vi "Instrument Manager_CleanUp.vi"(8 "Error In":errorcluster) -> (0 "Error Out":errorcluster)   [LabVIEW 2024, in "Instrument Manager.lvclass"]
uses:
  Instrument Manager.lvclass
  Interfaces/IUnmanaged/IUnmanaged.lvclass
  Interfaces/IInstrument/IInstrument.lvclass
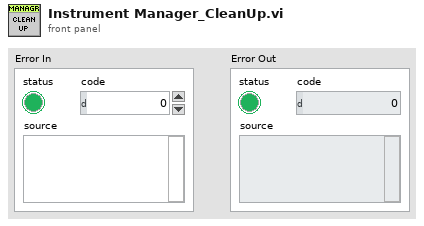
[diagram p1: front panel]
types:
  T1 = typedef "Instrument Manager.lvclass/ObjectAttributes.ctl" = cluster{"IInstruments":map{string, refnum<class "IInstrument.lvclass">}, "Instrument Configurations":map{string, refnum<class "Config from JSON.lvclass">}, "IVirtual Instruments":map{string, refnum<class "IVirtual Instrument.lvclass">}, "Virtual Instrument Configurations":map{string, refnum<class "Config from JSON.lvclass">}}
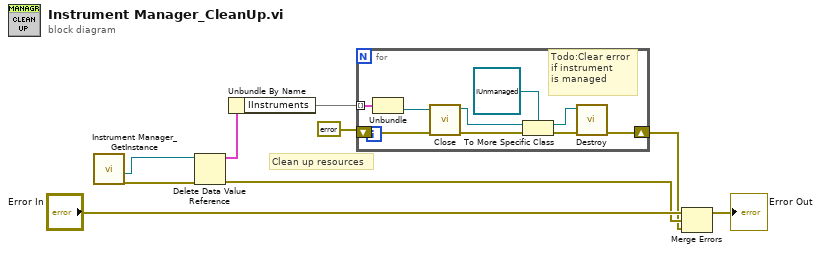
[diagram p0: block diagram]
diagram:
  # "Clean up resources"
  n1 = call "Instrument Manager_GetInstance.vi"() -> ("Error Out"=w5:errorcluster, "DVRRefOut"=w6:refnum<data-value>)  [unwired: 7 in, 3 out]
  n2 = Delete Data Value Reference(data value reference=w6, error in=w5) -> (data value=w4:T1, error out=w7:errorcluster)
  n3 = Unbundle By Name(w4) -> ("IInstruments"=w3:map{string, refnum<class "IInstrument.lvclass">})
  n4 = for {
    tunnel: w3 -> [w18] mode=indexing
    shift-right: [w13] -> w1
    shift-left: errorcluster {"status"=FALSE, "code"=0, "source"=""} ("error constant") -> [w15]
    # "Todo:Clear error\nif instrument\nis managed"
    n5 = Unbundle(w18) -> ("IInstrument"=w17:refnum<class "IInstrument.lvclass">)  [unwired: 1 out]
    n6 = call-dynamic "Close.vi"("error in"=w15, "IClose in"=w17) -> ("error out"=w16:errorcluster, "IClose out"=w10:refnum<class "IInstrument.lvclass">)  [unwired: 8 in]
    n7 = To More Specific Class(target class=refnum<class "IUnmanaged.lvclass"> refnum ("IUnmanaged.lvclass"), reference=w10, error in=w16) -> (specific class reference=w12:refnum<class "IUnmanaged.lvclass">, error out=w14:errorcluster)
    n8 = call-dynamic "Destroy.vi"("error in"=w14, "IUnmanaged in"=w12) -> ("error out"=w13:errorcluster)  [unwired: 8 in, 1 out]
  }
  n9 = Merge Errors("Error In", w7, w1) -> (→"Error Out":errorcluster)
